vi "Get_Measurements.vi"(0 "VISA resource name":refnum<visa-resource-name>="Oscilloscope", 2 "Delay_Index":i32, 4 "Measurements per channel":i32=5, 6 "Amplitude":bool=TRUE, 7 "file path (dialog if empty)":path=path "F:/L0_Measurements_291014_174904.txt", 8 "Width":bool=TRUE, 9 "Write to a file?":bool, 10 "Delay_Line_Number":i32, 11 "error in":errorcluster, 12 "Delay":bool=TRUE, 13 "Oscilloscope Channel":i32(ring)=1 items=["Channel 1"=1, "Channel 2"=2, "Channel 3"=3, "Channel 4"=4, "Function 1"=5, "Function 2"=6, "Function 3"=7, "Function 4"=8, "Memory 1"=9, "Memory 2"=10, "Memory 3"=11, "Memory 4"=12]) -> (14 "VISA resource name out":refnum<visa-resource-name>="Oscilloscope", 15 "Vpp_Array":dbl[](array[numeric]), 16 "Width Array":dbl[](array[numeric]), 18 "Setup_Time_Array":dbl[](array[numeric]), 19 "error out":errorcluster)   [LabVIEW 2009]
uses:
  <vilib>/Utility/file.llb/Write To Spreadsheet File (string).vi
panel:
  in  "Delay_Value":dbl[](array[numeric])=[0.0, 0.25, 0.5, 0.75, 1.0, 1.25, 1.5, 1.75, 2.0, 2.25, 2.5, 2.75, 3.0, 3.25, 3.5, 3.75, 4.0, 4.25, 4.5, 4.75, 5.0, 5.25, 5.5, 5.75, 2.0, 2.25, 2.5, 2.75, 3.0, 3.25, 3.5, 3.75]
  out "new file path (Not A Path if cancelled)":path=path "F:/L0_Measurements_291014_174904.txt"
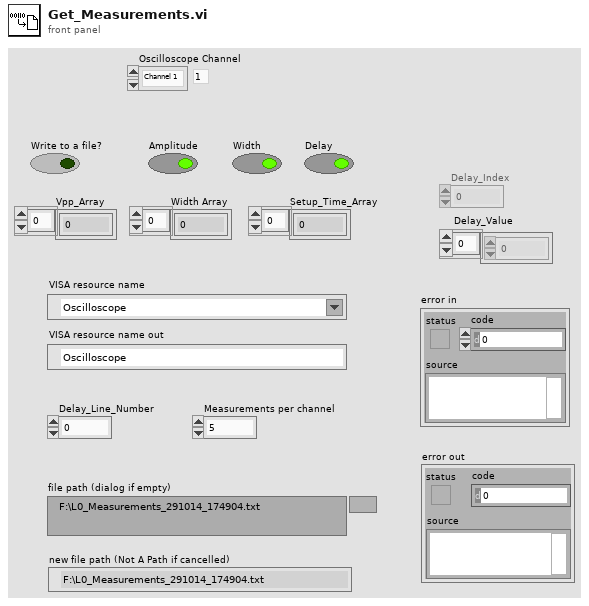
[diagram p1: front panel]
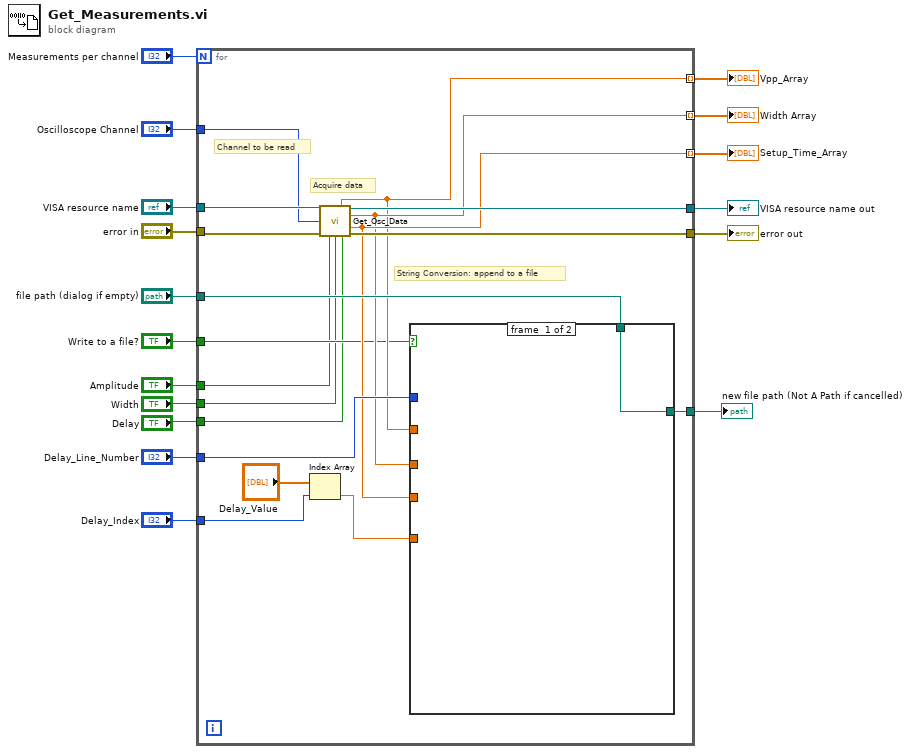
[diagram p0: block diagram]
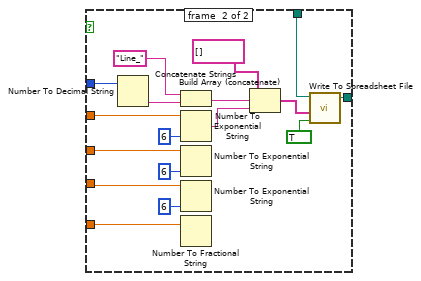
[diagram p2: hidden frame]
diagram:
  n1 = for {
    N: "Measurements per channel" -> [_]
    tunnel: "VISA resource name" -> [w35]
    tunnel: "error in" -> [w34]
    tunnel: "Delay_Line_Number" -> [w27]
    tunnel: "file path (dialog if empty)" -> [w29]
    tunnel: [w33] -> w12
    tunnel: [w32] -> w8
    tunnel: [w28] -> w11
    tunnel: "Delay_Index" -> [w30]
    tunnel: [w24] -> w9 mode=indexing
    tunnel: [w25] -> w7 mode=indexing
    tunnel: [w26] -> w6 mode=indexing
    tunnel: "Write to a file?" -> [w23]
    tunnel: "Amplitude" -> [w22]
    tunnel: "Width" -> [w21]
    tunnel: "Delay" -> [w20]
    tunnel: "Oscilloscope Channel" -> [w19]
    # "Acquire data"
    # "Channel to be read"
    # "String Conversion: append to a file"
    n2 = Index Array(array="Delay_Value", index=w30) -> (element=w18:dbl)
    n3 = call "Get_Osc_Data.vi"("VISA resource name"=w35, "Channel"=w19, "error in"=w34, "Amplitude"=w22, "Width"=w21, "Delay"=w20) -> ("Amplitude"=w24:dbl, "VISA resource name out"=w33:refnum<visa-resource-name>, "Width Pos"=w25:dbl, "Delay"=w26:dbl, "error out"=w32:errorcluster)  [unwired: 4 in, 1 out]
    n4 = case shown="True" w23 {
      tunnel: w29 -> [w36 w44]
      tunnel: [w36 w43] -> w28
      tunnel: w27 -> [_ w42]
      tunnel: w26 -> [_ w41]
      tunnel: w18 -> [_ w38]
      tunnel: w25 -> [_ w40]
      tunnel: w24 -> [_ w39]
      frame #0 {
      }
      frame #1 {
        n5 = Number To Decimal String(number=w42) -> (decimal integer string=w50:string)  [unwired: 1 in]
        n6 = Concatenate Strings("Line_", w50) -> (w48:string)
        n7 = Number To Exponential String(number=w39, precision (6)=i16 6) -> (E-format string=w37:string)  [unwired: 2 in]
        n8 = Number To Exponential String(number=w40, precision (6)=i16 6) -> ()  [unwired: 2 in, 1 out]
        n9 = Number To Exponential String(number=w41, precision (6)=i16 6) -> ()  [unwired: 2 in, 1 out]
        n10 = Number To Fractional String(number=w38) -> ()  [unwired: 3 in, 1 out]
        n11 = Build Array (concatenate)(string[] [] ("array"), w48, w37) -> (w52:string[])
        n12 = call-poly <vilib>:"Write To Spreadsheet File.vi"("append to file? (new file:F)"=TRUE, "1D data"=w52, "file path (dialog if empty)"=w44) -> ("new file path (Not A Path if cancelled)"=w43:path)  [unwired: 5 in]
      }
    }
  }
  "VISA resource name out" <- w12
  "error out" <- w8
  "new file path (Not A Path if cancelled)" <- w11
  "Vpp_Array" <- w9
  "Width Array" <- w7
  "Setup_Time_Array" <- w6
